vi "ErrorType.vi"(4 "Error in":errorcluster) -> (1 "Error type":T1)   [LabVIEW 2017, in "GPError.lvlib"]
doc: "Determines the <B>Error type</B> of <B>Error in</B>.\n\nOrdinary (single-error) error clusters can be of <B>Error type</B> 'No error', 'Error', or 'Warning'.\n\nAppended errors can be of <B>Error type</B> 'Appended errors' (all errors), 'Appended warnings' (all warnings), or 'Appended mixed' (both errors and warnings).\n\nA warning uses the standard definition of Status being False while Code being non-zero.\n\nThis VI is inlined.\n\nSteen Schmidt\nGPower\n15/7 2013"
uses:
  GPError.lvlib
  Typedefs/ErrorType.ctl
panel:
  # "Copyright © 2014\nGPower\nSee enclosed license file for terms and conditions"
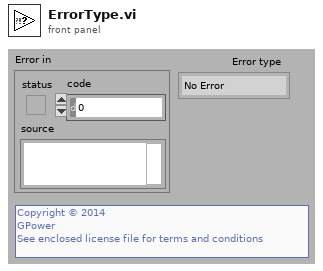
[diagram p1: front panel]
types:
  T1 = typedef "GPError.lvlib/ErrorType.ctl" = enum16{"No Error", "Error", "Warning", "Appended errors", "Appended warnings", "Appended mixed"}
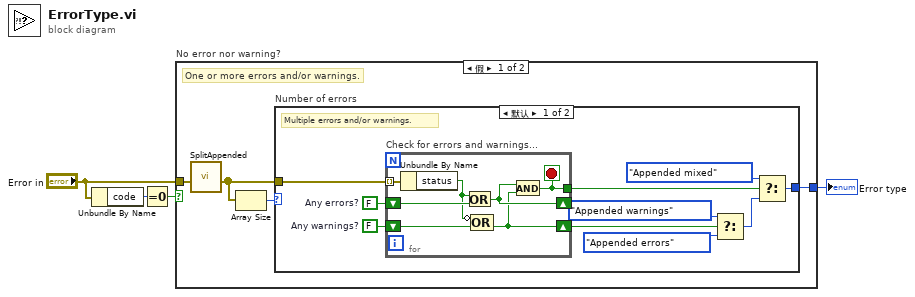
[diagram p0: block diagram]
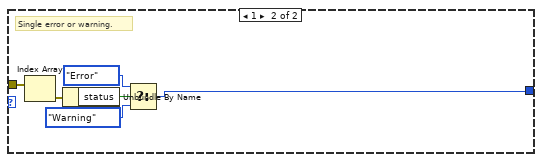
[diagram p2: hidden frame]
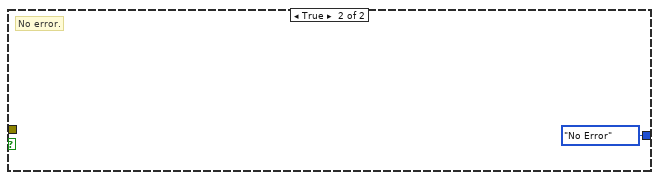
[diagram p3: hidden frame]
diagram:
  n1 = Unbundle By Name("Error in") -> ("code"=w4:i32)
  n2 = Equal To 0?(x=w4) -> (x = 0?=w2:bool)
  n3 = case "No error nor warning?" shown="假" w2 {
    tunnel: "Error in" -> [w8 _]
    tunnel: [w5 ErrorType."No Error" ("Error type")] -> w1
    frame False {
      # "One or more errors and/or warnings."
      n4 = call "SplitAppended.vi"("Appended errors in"=w8) -> ("Errors out"=w6:errorcluster[])  [unwired: 10 in]
      n5 = Array Size(array=w6) -> (size(s)=w7:i32)
      n6 = case "Number of errors" shown="默认" w7 {
        tunnel: w6 -> [w18 w31]
        tunnel: [w9 w26] -> w5
        frame Default {
          w16 = FALSE  # Any warnings?
          w17 = FALSE  # Any errors?
          # "Multiple errors and/or warnings."
          n7 = for "Check for errors and warnings..." {
            tunnel: w18 -> [w25] mode=indexing
            shift-right: [w21] -> _
            shift-left: w17 -> [w24]
            shift-right: [w20] -> w13
            shift-left: w16 -> [w23]
            tunnel: [w19] -> w15
            stop <- w19 stop-if-true
            n8 = Unbundle By Name(w25) -> ("status"=w22:bool)
            n9 = Or(x=w22, y=w24) -> (x .or. y?=w21:bool)
            n10 = Compound Arithmetic op=OR(invert w22, w23) -> (w20:bool)
            n11 = And(x=w21, y=w20) -> (x .and. y?=w19:bool)
          }
          n12 = Select(t=ErrorType."Appended warnings" ("Error type"), s=w13, f=ErrorType."Appended errors" ("Error type")) -> (s? t:f=w10:T1)
          n13 = Select(t=ErrorType."Appended mixed" ("Error type"), s=w15, f=w10) -> (s? t:f=w9:T1)
        }
        frame 1 {
          # "Single error or warning."
          n14 = Index Array(array=w31) -> (element=w30:errorcluster)  [unwired: 1 in]
          n15 = Unbundle By Name(w30) -> ("status"=w27:bool)
          n16 = Select(t=ErrorType."Error" ("Error type"), s=w27, f=ErrorType."Warning" ("Error type")) -> (s? t:f=w26:T1)
        }
      }
    }
    frame True {
      # "No error."
    }
  }
  "Error type" <- w1
